vi "Position Message String.vi"(8 "error in (no error)":errorcluster, 11 "String Ref":refnum<vi>) -> (0 "error out":errorcluster)   [LabVIEW 2014]
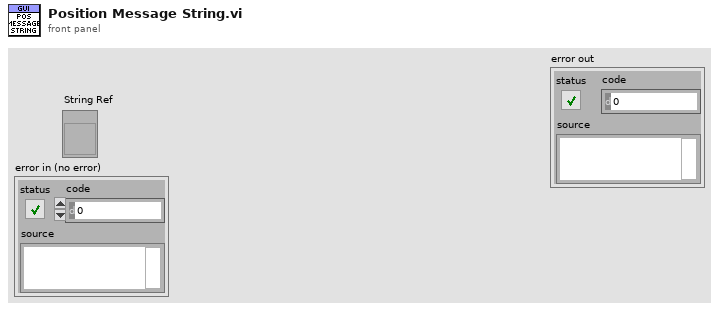
[diagram p1: front panel]
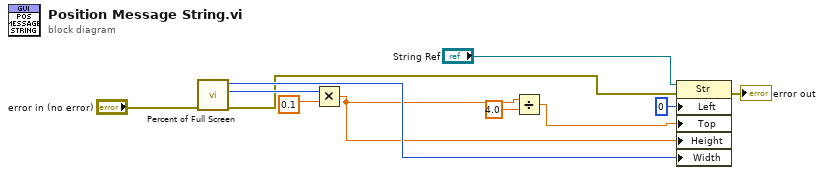
[diagram p0: block diagram]
diagram:
  n1 = call "Percent of Full Screen.vi"("error in (no error)"="error in (no error)") -> ("error out"=w5:errorcluster, "Bottom"=w8:i16, "Right"=w6:i16)  [unwired: 8 in]
  n2 = Multiply(x=w8, y=0.1) -> (x*y=w3:dbl)
  n3 = Divide(x=w3, y=4.0) -> (x/y=w1:dbl)
  n4 = property class="Str"(reference="String Ref", error in=w5, "Left"=0 ("Position:Left"), "Top"=w1, "Height"=w3, "Width"=w6) -> (error out=→"error out":errorcluster)  [unwired: 1 out]
